vi "getEposInCurrentUnits.vi"(8 "error in (no error)":errorcluster, 11 "Axis in":refnum<class "Axis.lvclass">) -> (0 "error out":errorcluster, 2 "EPOS In Current Units":dbl, 3 "Axis out":refnum<class "Axis.lvclass">)   [LabVIEW 2019, in "Axis.lvclass"]
uses:
  Axis.lvclass
  Axis.lvclass/Axis.ctl
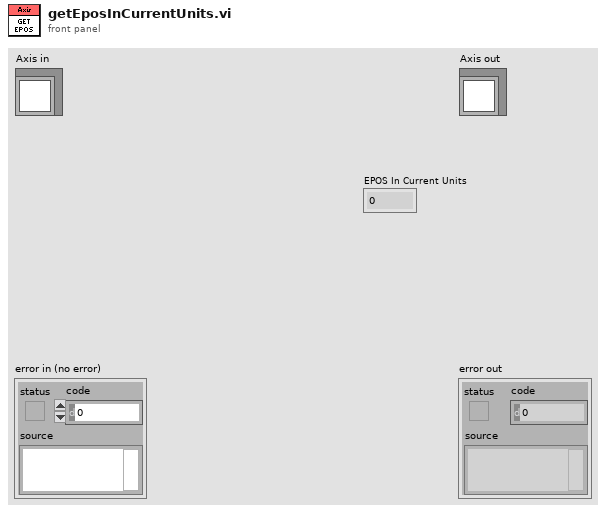
[diagram p1: front panel]
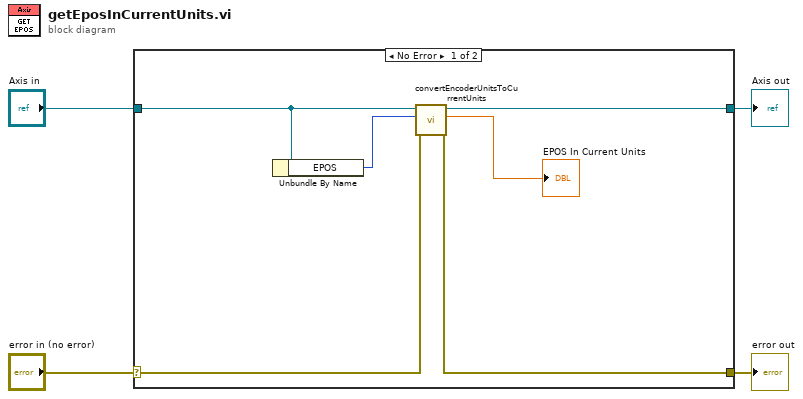
[diagram p0: block diagram]
diagram:
  n1 = case shown="No Error" "error in (no error)" {
    selector: "error in (no error)" -> [w7 w12]
    tunnel: [w6 w12] -> w3
    tunnel: [w9 w11] -> w1
    tunnel: "Axis in" -> [w10 w11]
    frame No Error {
      n2 = Unbundle By Name(w10) -> ("EPOS"=w8:i32)
      n3 = call-dynamic "convertEncoderUnitsToCurrentUnits.vi"("error in (no error)"=w7, "Value In Encoder Units"=w8, "Axis in"=w10) -> ("error out"=w6:errorcluster, "Value In Current Units"=→"EPOS In Current Units":dbl, "Axis out"=w9:refnum<class "Axis.lvclass">)  [unwired: 6 in]
    }
    frame Error {
    }
  }
  "error out" <- w3
  "Axis out" <- w1
